vi "Circle Spot Calculator.vi"(7 "Center Y":i32, 8 "Radius":i32, 9 "Center X":i32, 10 "initialized array":i32[][](array[numeric])) -> (3 "Array":i32[][](array[numeric]))   [LabVIEW 2016]
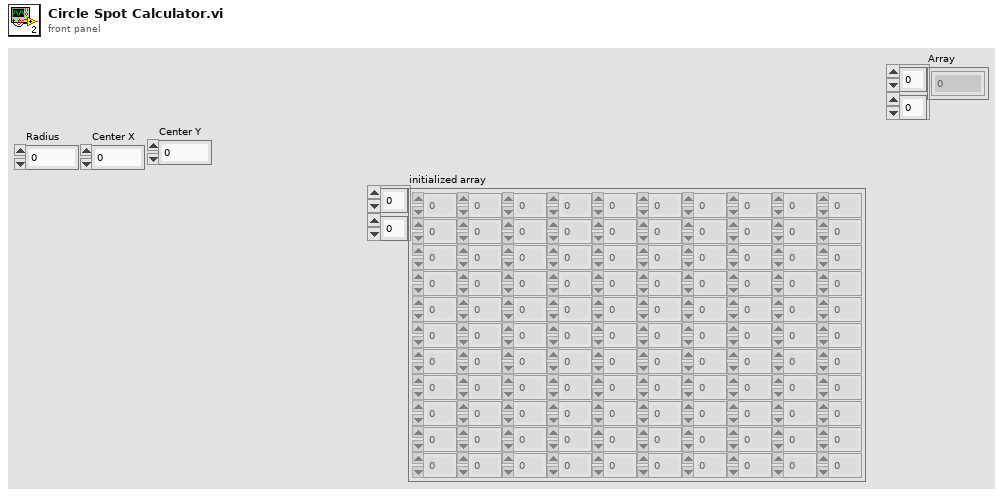
[diagram p1: front panel]
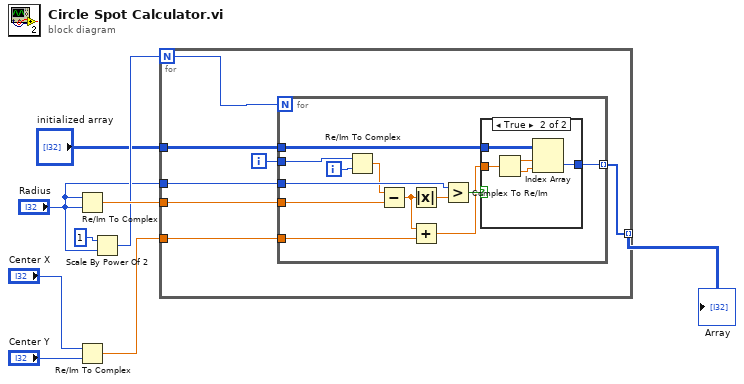
[diagram p0: block diagram]
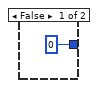
[diagram p2: hidden frame]
diagram:
  n1 = Re/Im To Complex(1:"Radius", 2:"Radius") -> (0:w8:cdb)
  n2 = Re/Im To Complex(1:"Center Y", 2:"Center X") -> (0:w7:cdb)
  n3 = Scale By Power Of 2(n=i16 1, x="Radius") -> (x*2^n=w5:i32)
  n4 = for {
    N: w5 -> [w16]
    tunnel: "initialized array" -> [w15]
    tunnel: "Radius" -> [w14]
    tunnel: w8 -> [w12]
    tunnel: w7 -> [w11]
    tunnel: [w10] -> w1 mode=indexing
    i -> [w13]
    n5 = for {
      N: w16 -> [_]
      tunnel: w15 -> [w21]
      tunnel: w14 -> [w28]
      tunnel: w13 -> [w26]
      tunnel: w12 -> [w22]
      tunnel: w11 -> [w18]
      tunnel: [w17] -> w10 mode=indexing
      i -> [w25]
      n6 = Re/Im To Complex(1:w25, 2:w26) -> (0:w24:cdb)
      n7 = Subtract(x=w24, y=w22) -> (x-y=w19:cdb)
      n8 = Absolute Value(x=w19) -> (abs(x)=w23:dbl)
      n9 = Add(x=w19, y=w18) -> (x+y=w20:cdb)
      n10 = Greater?(x=w28, y=w23) -> (0:w27:bool)
      n11 = case shown="True" w27 {
        tunnel: w21 -> [_ w34]
        tunnel: w20 -> [_ w33]
        tunnel: [0 w30] -> w17
        frame False {
        }
        frame True {
          n12 = Complex To Re/Im(x + iy=w33) -> (x=w31:dbl, y=w32:dbl)
          n13 = Index Array(array=w34, index (row)=w31, index (col)=w32) -> (element=w30:i32)
        }
      }
    }
  }
  "Array" <- w1
